vi "checkBeginDirectKickPlay.vi"(8 "error in (no error)":errorcluster, 10 "Game":refnum<class "Game.lvclass">, 11 "DirectKickPlay in":refnum<class "DirectKickPlay.lvclass">) -> (0 "error out":errorcluster, 2 "Boolean":bool, 3 "DirectKickPlay out":refnum<class "DirectKickPlay.lvclass">)   [LabVIEW 2023, in "DirectKickPlay.lvclass"]
uses:
  DirectKickPlay.lvclass
  Game_class/Game.lvclass
  Utilities_class/Utilities.lvclass
  Referee_class/command_interpreted.ctl
  Game_class/Game.lvclass/Game.ctl
  Referee_class/Referee.lvclass/Referee.ctl
  Game_class/Read Referee.vi
  Game_class/Read EventsRef.vi
  Referee_class/Read command_interpreted.vi
  Referee_class/Referee.lvclass
  Events_class/Events.lvclass
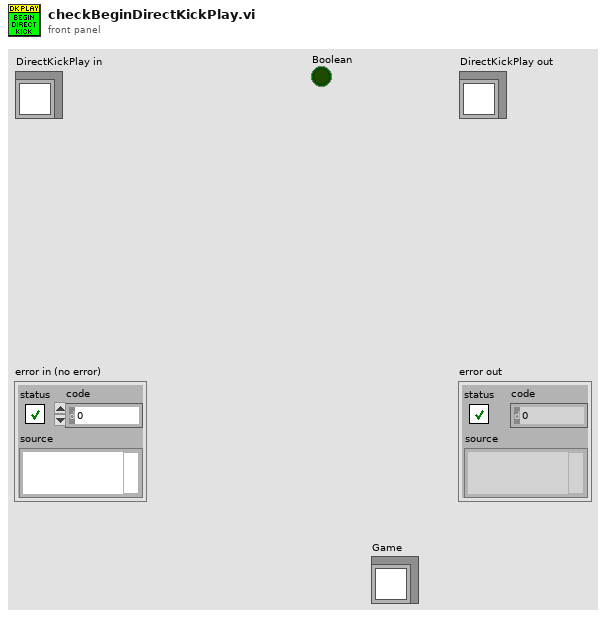
[diagram p1: front panel]
types:
  T1 = typedef "command_interpreted.ctl" = enum16{"Goal Ally", "Goal Enemy", "Ball Placement Enemy", "Ball Placement Ally", "Normal Half Time", "Extra Time  Break", "Extra Half Time", "None", "Post Game", "PKA Normal Start", "Prepare Kickoff Ally", "PKE Normal Start", "Prepare Kickoff Enemy", "Force Start", "Halt", "Timeout", "Prepare Penalty Ally", "Prepare Penalty Enemy", "PPA NormalStart", "PPE Normal Start", "Indirect Free Ally", "Direct Free Enemy", "Direct Free Ally", "Indirect Free Enemy", "Stop"}
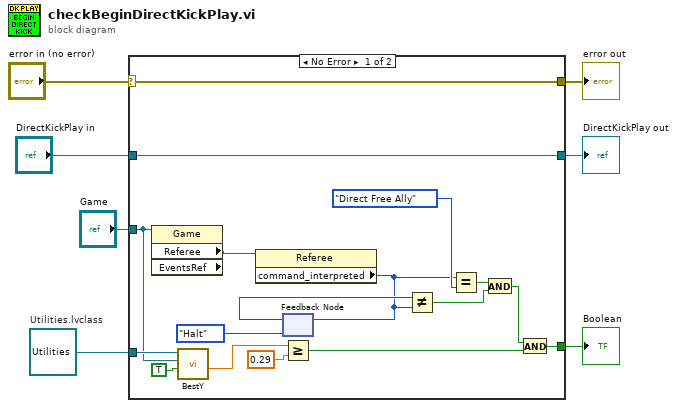
[diagram p0: block diagram]
diagram:
  w2 = refnum<class "Utilities.lvclass"> refnum  # Utilities.lvclass
  n1 = case shown="No Error" "error in (no error)" {
    selector: "error in (no error)" -> [w23 w26]
    tunnel: [w23 w26] -> w6
    tunnel: [w24 w25] -> w4
    tunnel: "DirectKickPlay in" -> [w24 w25]
    tunnel: "Game" -> [w14 _]
    tunnel: w2 -> [w15 _]
    tunnel: [w8 _] -> w1
    frame No Error {
      n2 = property class="Game" props=["Referee", "EventsRef"](reference=w14) -> ("Referee"=w22:refnum<class "Referee.lvclass">)  [unwired: 1 in, 3 out]
      n3 = call "BestY.vi"("Utilities in"=w15, "Game"=w14, "inimigos"=TRUE) -> ("Gap kick"=w12:dbl)  [unwired: 2 in, 4 out]
      n4 = property class="Referee"(reference=w22) -> ("command_interpreted"=w18:T1)  [unwired: 1 in, 2 out]
      n5 = feedback #1(command_interpreted."Halt" ("command_interpreted")) -> (w19:T1)
      n6 = feedback-in #1(w18) -> ()
      n7 = Greater Or Equal?(x=w12, y=0.29) -> (x >= y?=w10:bool)
      n8 = Not Equal?(x=w19, y=w18) -> (x != y?=w17:bool)
      n9 = Equal?(x=w18, y=command_interpreted."Direct Free Ally" ("command_interpreted")) -> (x = y?=w20:bool)
      n10 = And(x=w20, y=w17) -> (x .and. y?=w9:bool)
      n11 = And(x=w9, y=w10) -> (x .and. y?=w8:bool)
    }
    frame Error {
    }
  }
  "error out" <- w6
  "DirectKickPlay out" <- w4
  "Boolean" <- w1
